vi "task.active_lua.vi"(5 "LuaVIEW reference":T1) -> (15 "error out":errorcluster)   [LabVIEW 2012]
doc: "Set the task mode to \"running\" when launched asynchronously via \"Run Task\" or to \"executing\" when launched synchronously via \"Do Task\". When no \"--#defer\" preprocessor keyword is used, this is done automatically as soon as the main script starts to execute.\n\nThis function should be used when handling the resume signal or when the \"--#defer\" preprocessor keyword has left the task in \"initializing\" or \"swapping\" mode. Such deferred initialization allows the task to perform some additional initialization. Once a task is no longer \"initializing\" and the task is launched asynchronously, \"Run Task\" will return. This prevents the launching context from proceeding before requisite initialization actions are complete or subsequently required resources are allocated.\nErrors:\nFunction must be called from a task context but was not."
uses:
  typedefs/t_LuaVIEW Reference.ctl
  typedefs/t_LuaVIEW Task State Methods.ctl
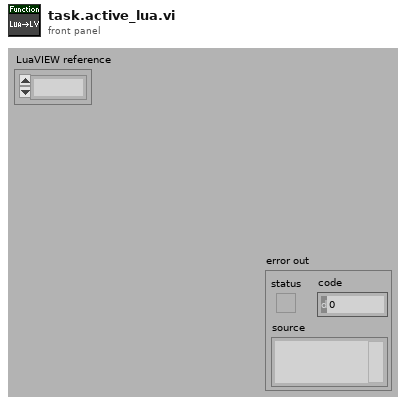
[diagram p1: front panel]
types:
  T1 = typedef "t_LuaVIEW Reference.ctl" = refnum<k1>
  T2 = typedef "t_LuaVIEW Task State Methods.ctl" = enum16{"cleanup", "set initial", "set mode", "set active mode", "set error", "get task info", "get script info", "set signal", "clear signal", "test handled", "test delegated", "test signal", "handle signal", "delegate signal", "allow signal", "disallow signal", "disallow all", "signals?", "delegated signals?", "protection++", "protection--", "protection=0", "message", "next message", "pop message", "message available?", "force stop", "set swap preps", "apply swap preps"}
  T3 = typedef "t_LuaVIEW Task State Pane.ctl" = refnum<vi>
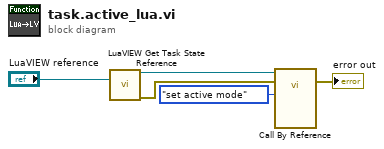
[diagram p0: block diagram]
diagram:
  n1 = call "LuaVIEW Get Task State Reference.vi"("LuaVIEW reference in"="LuaVIEW reference") -> ("task state reference"=w3:T3, "error out"=w2:errorcluster)  [unwired: 12 in, 1 out]
  n2 = call-by-ref "?"(reference=w3, error in=w2, "method"=t_LuaVIEW_Task_State_Methods."set active mode") -> (error out=→"error out":errorcluster)  [unwired: 10 in, 6 out]
